vi "XYZ Stage Driver.vi"(11 "UI elements cluster":T1) -> (0 "error out (no error)":errorcluster)   [LabVIEW 2013]
uses:
  Typedefs/XYZ stage states.ctl
  Typedefs/UI ctrl refs cluster.ctl
  Typedefs/Laser control knob.ctl
  Typedefs/Frame Size.ctl
  Typedefs/Plane Mode.ctl
  Typedefs/PMT control knob.ctl
  Typedefs/HW config states enum.ctl
  Globals/gl_XYZStage globals.vi
  Global Variables/General Globals.vi
  Global Variables/gl_UI Ctrl Refs.vi
panel:
  out "Command":T2
  out "Coordinates":cluster{"X":sgl, "Y":sgl, "Z":sgl}
  out "internal error cluster":errorcluster
  # "XYZ STAGE DRIVER"
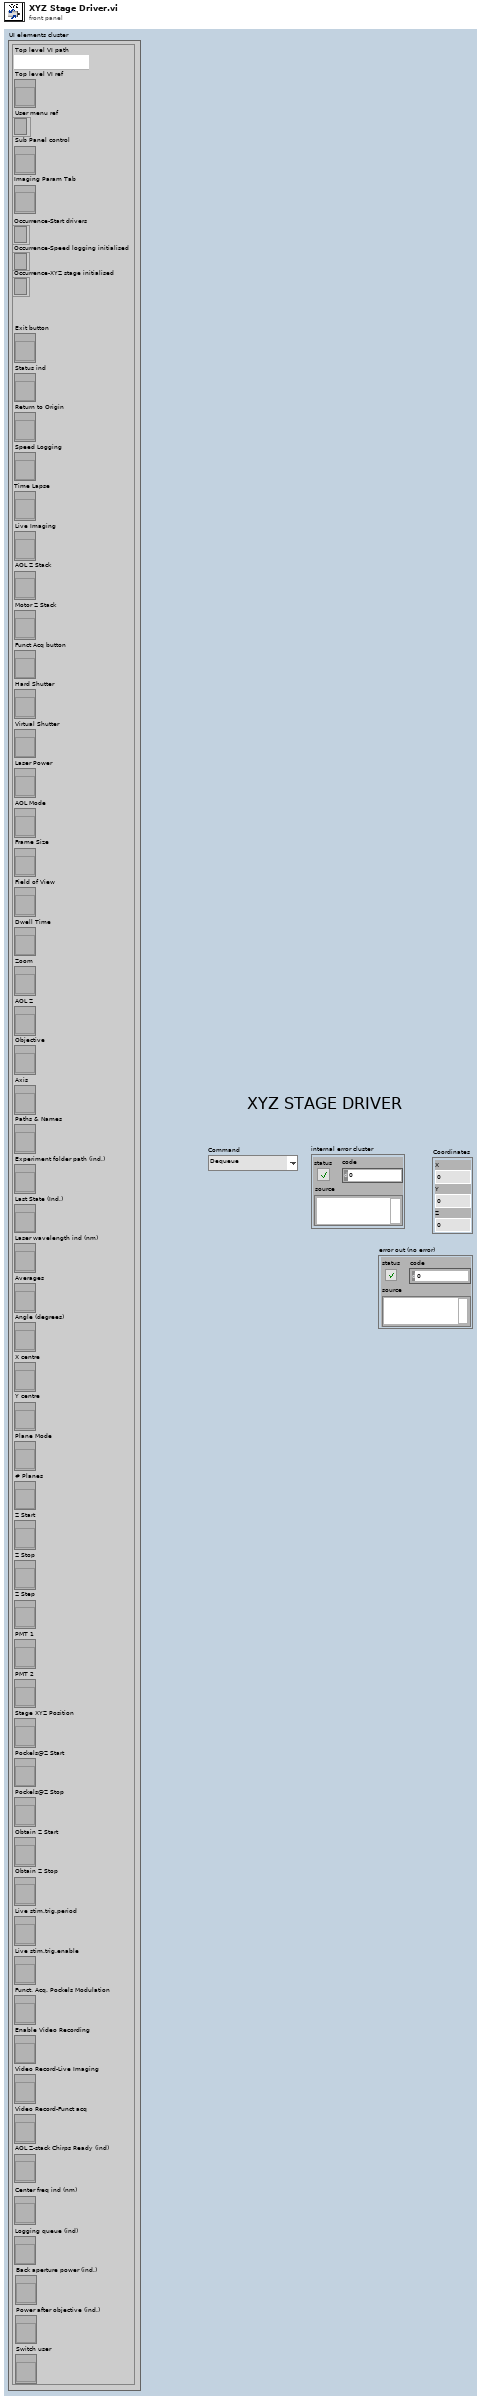
[diagram p1: front panel]
types:
  T1 = typedef "UI ctrl refs cluster.ctl" = cluster{"Top level VI path":path, "Top level VI ref":refnum<vi>, "User menu ref":refnum<k9>, "Sub Panel control":refnum<vi>, "Imaging Param Tab":refnum<vi>, "Occurrence-Start drivers":refnum<k4>, "Occurrence-Speed logging initialised":refnum<k4>, "Occurrence-XYZ stage initialised":refnum<k4>, "Exit button":refnum<vi>, "Status ind":refnum<vi>, "Return to Origin":refnum<vi>, "Speed Logging":refnum<vi>, "Time Lapse":refnum<vi>, "Live Imaging":refnum<vi>, "AOL Z Stack":refnum<vi>, "Motor Z Stack":refnum<vi>, "Funct Acq button":refnum<vi>, "Hard Shutter":refnum<vi>, "Virtual Shutter":refnum<vi>, "Laser Power":refnum<vi>, "AOL Mode":refnum<vi>, "Frame Size":refnum<vi>, "Field of View":refnum<vi>, "Dwell Time":refnum<vi>, "Zoom":refnum<vi>, "AOL Z":refnum<vi>, "Objective":refnum<vi>, "Axis":refnum<vi>, "Paths & Names":refnum<vi>, "Experiment folder path (ind.)":refnum<vi>, "Last State (Ind.)":refnum<vi>, "Laser wavelength ind (nm)":refnum<vi>, "Averages":refnum<vi>, "Angle (degrees)":refnum<vi>, "X centre":refnum<vi>, "Y centre":refnum<vi>, "Plane Mode":refnum<vi>, "# Planes":refnum<vi>, "Z Start":refnum<vi>, "Z Stop":refnum<vi>, "Z Step":refnum<vi>, "PMT 1":refnum<vi>, "PMT 2":refnum<vi>, "Stage XYZ Position":refnum<vi>, "Pockels@Z Start":refnum<vi>, "Pockels@Z Stop":refnum<vi>, "Obtain Z Start":refnum<vi>, "Obtain Z Stop":refnum<vi>, "Live stim.trig.period":refnum<vi>, "Live stim.trig.enable":refnum<vi>, "Funct. Acq. Pockels Modulation":refnum<vi>, "Enable Video Recording":refnum<vi>, "Video Record-Live Imaging":refnum<vi>, "Video Record-Funct acq":refnum<vi>, "AOL Z-stack Chirps Ready (ind)":refnum<vi>, "Center freq ind (nm)":refnum<vi>, "Logging queue (ind)":refnum<vi>, "Back aperture power (ind.)":refnum<vi>, "Power after objective (ind.)":refnum<vi>, "Switch user":refnum<vi>}
  T2 = typedef "XYZ stage states.ctl" = enum16{"Dequeue", "Initialize", "Read Position", "Read Speed Setting", "Move", "Set Max Speed", "Reset Axis", "Stop all movement"}
  T3 = typedef "HW config states enum.ctl" = enum16{"Load from file", "Save to file", "Write all", "Read all", "Write XY stage settings", "Write DAQ FPGA settings", "Write Control FPGA settings", "Write Phys Channels", "Clear", "Compare from file"}
  T4 = typedef "Sys Configuration.ctl" = cluster{"XY Stage":T5, "DAQ FPGA":T6, "Control system":T10, "Encoder":T11, "DAQmx Chan":T12, "Computer MAC address":string, "Cam VidRec":T13, "Externalise Triggers":bool, "Laser wavelength (nm)":dbl}
  T5 = typedef "XY Stage config cluster.ctl" = cluster{"COM port":refnum<visa-resource-name>, "XY stage available":bool}
  T6 = typedef "DAQ FPGA config cluster.ctl" = cluster{"Ref":T7, "Target":T8, "Clock Freq (MHz) ":dbl, "input card type":T9, "Samples Wait after Trigger":u16, "AOD fill":u16, "StartupDelay":i32, "Slip Cycle (clock cycles)":u32, "Add Cycle":bool}
  T7 = typedef "FPGA Ref.ctl" = refnum<k20>
  T8 = typedef "nirio_resource_hc.ctl" = tag
  T9 = typedef "FPGA input type AC-DC.ctl" = enum16{"AC Card", "DC Card"}
  T10 = typedef "CTRL system config cluster.ctl" = cluster{"Ethernet opened":bool, "Ethernet Port":u32, "Ctrl FPGA available":bool, "Ctrl FPGA Clock (MHz)":dbl, "Ctrl system MAC address":string, "Control system.Network adapter name":string, "AOD 1 Amplitude":i16, "AOD 2 Amplitude":i16, "AOD 3 Amplitude":i16, "AOD 4 Amplitude":i16, "Data Time Interval (ns)":dbl, "T0 (ns)":dbl, "Ta (ns)":dbl}
  T11 = typedef "Encoder config cluster.ctl" = cluster{"IP address":string, "Port":u16, "Encoder available":bool, "Wheel radius (cm)":dbl}
  T12 = typedef "DAQmx physical channels cluster.ctl" = cluster{"Pockels AO":tag, "Hard shutter AO":tag, "PMT AOs":tag, "Power meter AI":tag}
  T13 = typedef "Cam VidRec HW config setup cluster.ctl" = cluster{"DO flag-Video record":tag, "DO flag-Trial start":tag, "VidRec available":bool}
  T14 = typedef "XYZ stage data.ctl" = cluster{"Command":T2, "Channel":T15, "X":sgl, "Y":sgl, "Z":sgl, "Speed":i32, "Zero":bool, "Use acknowledgement?":bool}
  T15 = typedef "XYZ channel ring.ctl" = string
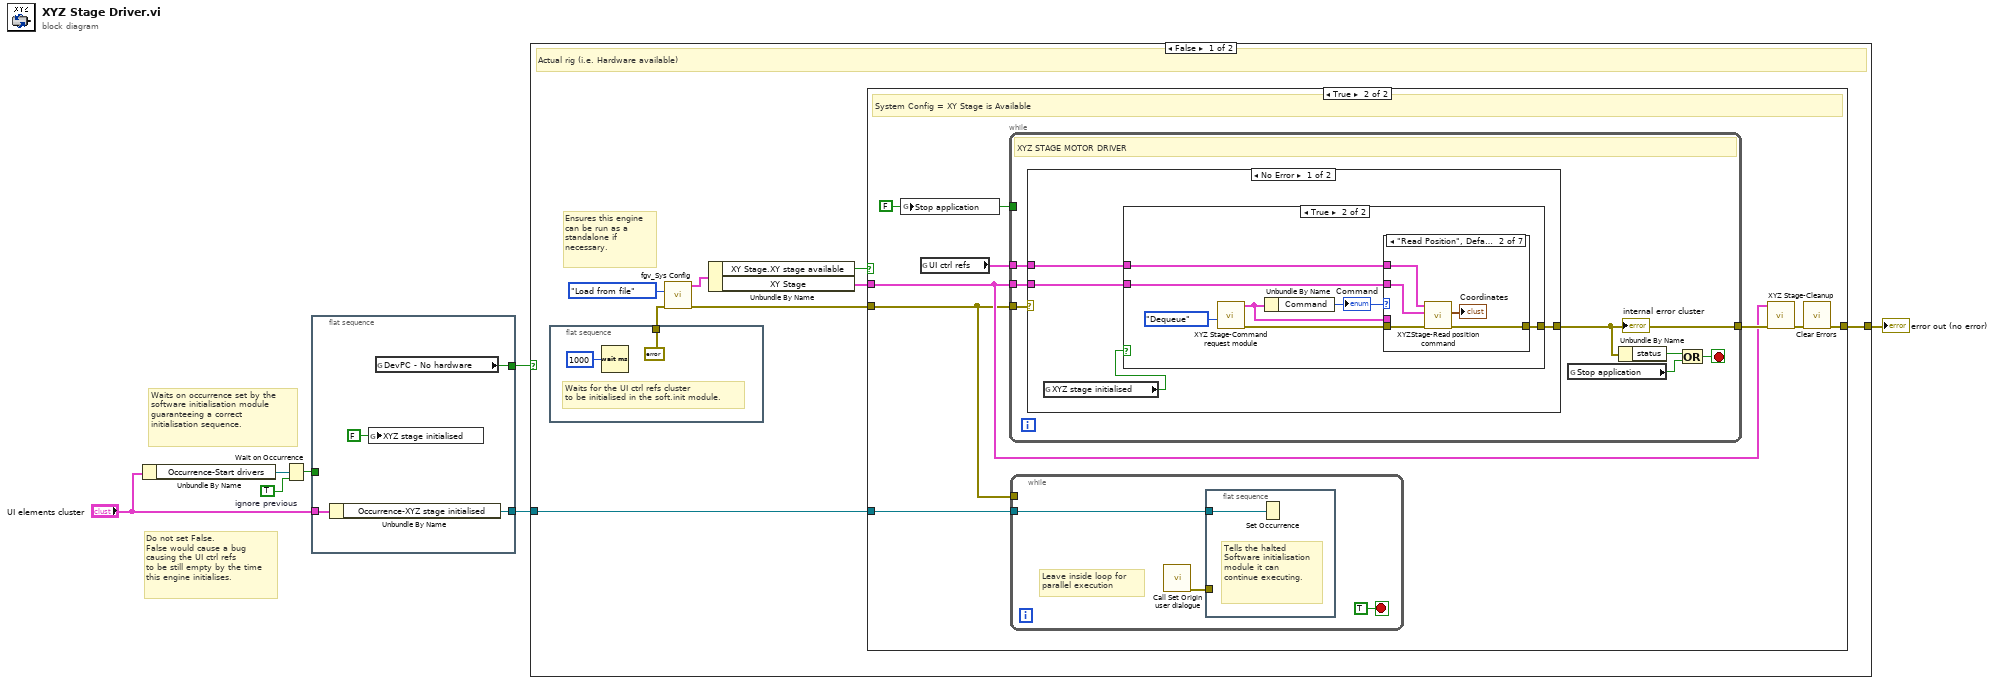
[diagram p0: block diagram]
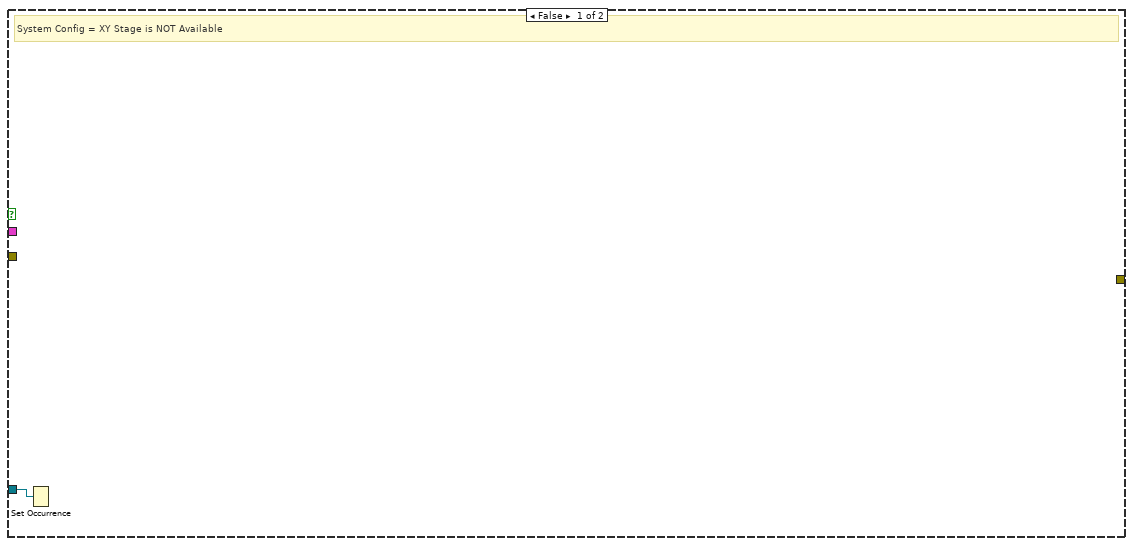
[diagram p2: hidden frame]
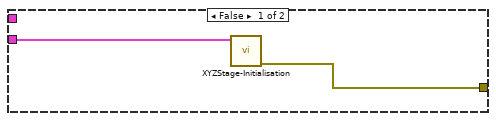
[diagram p3: hidden frame]
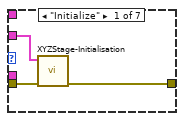
[diagram p4: hidden frame]
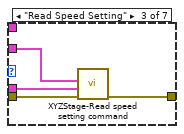
[diagram p5: hidden frame]
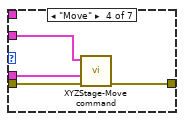
[diagram p6: hidden frame]
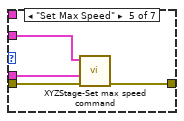
[diagram p7: hidden frame]
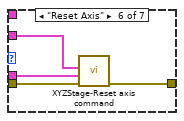
[diagram p8: hidden frame]
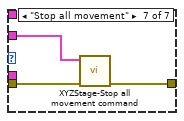
[diagram p9: hidden frame]
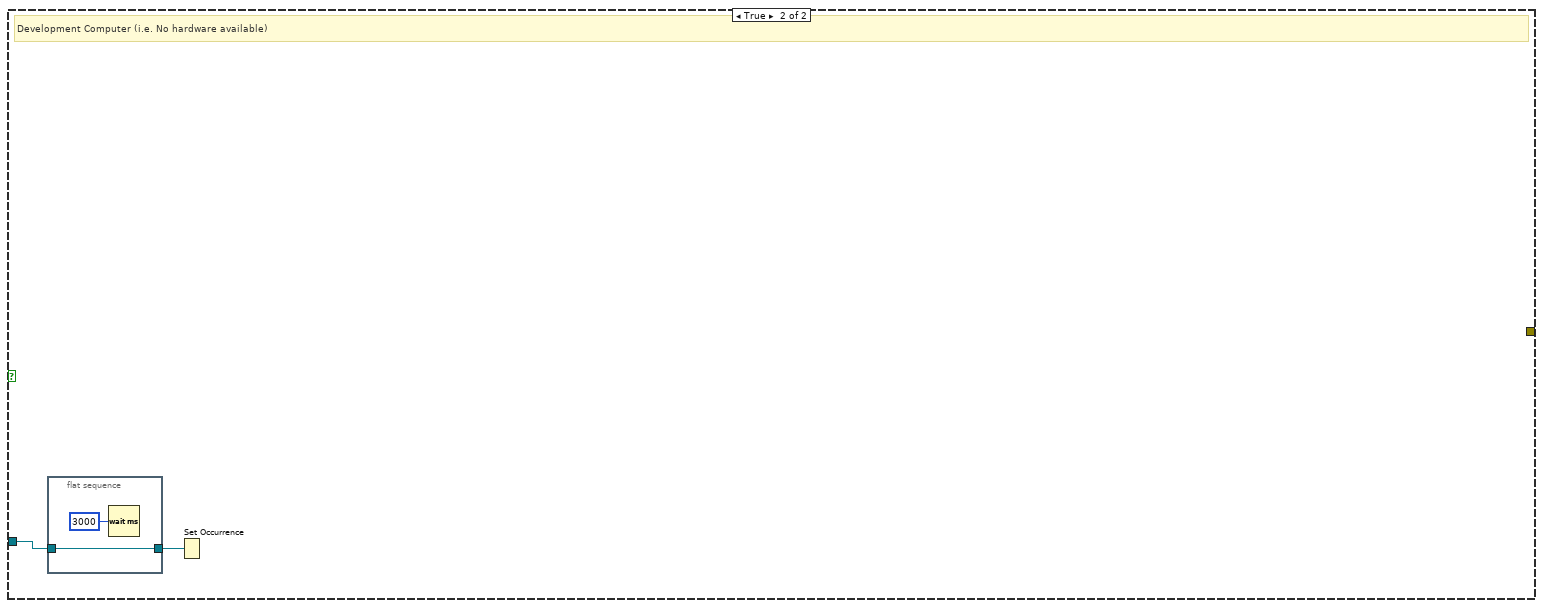
[diagram p11: hidden frame]
diagram:
  w3 = TRUE  # ignore previous
  # "Do not set False.\nFalse would cause a bug\ncausing the UI ctrl refs\nto be still empty by the time\nthis engine initialises."
  # "Waits on occurrence set by the software initialisation module guaranteeing a correct initialisation sequence."
  n1 = Unbundle By Name("UI elements cluster") -> ("Occurrence-Start drivers"=w2:refnum<k4>)
  n2 = Wait on Occurrence(1:w3, 2:w2) -> (0:w1:bool)  [unwired: 1 in]
  n3 = flat-sequence {
    tunnel: [w11] -> w6
    tunnel: "UI elements cluster" -> [w10]
    tunnel: [w9] -> w5
    tunnel: w1 -> [_]
    frame #0 {
      n4 = Unbundle By Name(w10) -> ("Occurrence-XYZ stage initialised"=w9:refnum<k4>)
      n5 = global write "gl_XYZStage globals.vi" "XYZ stage initialised"(FALSE ("XYZ stage initialised")) -> ()
      n6 = global read "General Globals.vi" "DevPC - No hardware"() -> (w11:bool)
    }
  }
  n7 = case shown="False" w6 {
    tunnel: [w15 _] -> w7
    tunnel: w5 -> [w12 w84]
    frame False {
      # "Ensures this engine can be run as a standalone if necessary."
      # "Actual rig (i.e. Hardware available)"
      n8 = flat-sequence {
        tunnel: [errorcluster {"status"=FALSE, "code"=0, "source"=""} ("error in (no error)")] -> w13
        frame #0 {
          # "Waits for the UI ctrl refs cluster\nto be initialised in the soft.init module."
          n9 = Wait (ms)(milliseconds to wait=u32 1000) -> ()  [unwired: 1 out]
        }
      }
      n10 = call "fgv_Sys Config.vi"("error in (no error)"=w13, "Function"=HW_config_states_enum."Load from file") -> ("error out"=w16:errorcluster, "System Config out"=w17:T4)  [unwired: 8 in]
      n11 = Unbundle By Name(w17) -> ("XY Stage.XY stage available"=w14:bool, "XY Stage"=w19:T5)
      n12 = case shown="True" w14 {
        tunnel: w19 -> [_ w29]
        tunnel: w12 -> [w22 w28]
        tunnel: w16 -> [_ w26]
        tunnel: [_ w24] -> w15
        frame False {
          # "System Config = XY Stage is NOT Available"
          n13 = Set Occurrence(w22) -> ()
        }
        frame True {
          w27 = FALSE ("Stop application")
          # "System Config = XY Stage is Available"
          n14 = global write "General Globals.vi" "Stop application"(w27) -> ()
          n15 = global read "gl_UI Ctrl Refs.vi" "UI ctrl refs"() -> (w23:T1)
          n16 = while {
            tunnel: w26 -> [w38]
            tunnel: [w36] -> w30
            tunnel: w29 -> [w39]
            tunnel: w27 -> [_]
            tunnel: w23 -> [w35]
            stop <- w41 stop-if-true
            # "XYZ STAGE MOTOR DRIVER"
            n17 = case shown="No Error" w38 {
              selector: w38 -> [_ w82]
              tunnel: [w44 w82] -> w36
              tunnel: w39 -> [w45 _]
              tunnel: w35 -> [w42 _]
              frame No Error {
                n18 = global read "gl_XYZStage globals.vi" "XYZ stage initialised"() -> (w43:bool)
                n19 = case shown="True" w43 {
                  tunnel: w45 -> [w47 w54]
                  tunnel: [w46 w53] -> w44
                  tunnel: w42 -> [_ w48]
                  frame False {
                    n20 = call "XYZStage-Initialisation.vi"("XY Stage"=w47) -> ("Error Out"=w46:errorcluster)  [unwired: 9 in, 1 out]
                  }
                  frame True {
                    n21 = call "XYZ Stage-Command request module.vi"("Command"=XYZ_stage_states."Dequeue") -> ("error out"=w51:errorcluster, "XYZ Stage dequeued data"=w50:T14)  [unwired: 6 in, 3 out]
                    n22 = Unbundle By Name(w50) -> ("Command"=w52:T2)
                    "Command" <- w52
                    n23 = case shown="\"Read Position\", Default" w52 {
                      tunnel: w54 -> [w56 w61 w66 w68 w72 w78 w79]
                      tunnel: w50 -> [_ _ w63 w67 w71 w75 _]
                      tunnel: w51 -> [w57 w62 w65 w70 w74 w76 w80]
                      tunnel: [w55 w60 w64 w69 w73 w77 w81] -> w53
                      tunnel: w48 -> [_ w58 _ _ _ _ _]
                      frame "Initialize" {
                        n24 = call "XYZStage-Initialisation.vi"("Error In"=w57, "XY Stage"=w56) -> ("Error Out"=w55:errorcluster)  [unwired: 8 in, 1 out]
                      }
                      frame "Read Position", Default {
                        n25 = call "XYZStage-Read position command.vi"("error in (no error)"=w62, "XY Stage config cluster"=w61, "UI ctrl refs"=w58) -> ("error out"=w60:errorcluster, "Coordinates"=→"Coordinates":cluster{"X":sgl, "Y":sgl, "Z":sgl})  [unwired: 7 in]
                      }
                      frame "Read Speed Setting" {
                        n26 = call "XYZStage-Read speed setting command.vi"("error in (no error)"=w65, "XYZ Stage data to queue"=w63, "XY Stage config cluster"=w66) -> ("error out"=w64:errorcluster)  [unwired: 8 in]
                      }
                      frame "Move" {
                        n27 = call "XYZStage-Move command.vi"("Error In"=w70, "XYZ Stage data"=w67, "XYZ Stage config"=w68) -> ("Error Out"=w69:errorcluster)  [unwired: 7 in, 1 out]
                      }
                      frame "Set Max Speed" {
                        n28 = call "XYZStage-Set max speed command.vi"("Error In"=w74, "XYZ Stage data"=w71, "XYZ Stage config"=w72) -> ("Error Out"=w73:errorcluster)  [unwired: 8 in]
                      }
                      frame "Reset Axis" {
                        n29 = call "XYZStage-Reset axis command.vi"("error in (no error)"=w76, "XYZ Stage dequeued data"=w75, "XY Stage"=w78) -> ("error out"=w77:errorcluster)  [unwired: 8 in]
                      }
                      frame "Stop all movement" {
                        n30 = call "XYZStage-Stop all movement command.vi"("Error In"=w80, "XYZ Stage config"=w79) -> ("Error Out"=w81:errorcluster)  [unwired: 8 in, 1 out]
                      }
                    }
                  }
                }
              }
              frame Error {
              }
            }
            "internal error cluster" <- w36
            n31 = global read "General Globals.vi" "Stop application"() -> (w37:bool)
            n32 = Unbundle By Name(w36) -> ("status"=w40:bool)
            n33 = Compound Arithmetic op=OR(w40, w37) -> (w41:bool)
          }
          n34 = while {
            tunnel: w26 -> [_]
            tunnel: w28 -> [w31]
            stop <- TRUE stop-if-true
            # "Leave inside loop for parallel execution"
            n35 = call "Call Set Origin user dialogue.vi"() -> ("error out"=w32:errorcluster)  [unwired: 11 in]
            n36 = flat-sequence {
              tunnel: w32 -> [_]
              tunnel: w31 -> [w34]
              frame #0 {
                # "Tells the halted Software initialisation\nmodule it can continue executing."
                n37 = Set Occurrence(w34) -> ()
              }
            }
          }
          n38 = call "XYZ Stage-Cleanup.vi"("error in (no error)"=w30, "XY Stage config cluster"=w29) -> ("error out"=w25:errorcluster)  [unwired: 9 in]
          n39 = call <vilib>:"Clear Errors.vi"("error in (no error)"=w25) -> ("error out"=w24:errorcluster)  [unwired: 6 in]
        }
      }
    }
    frame True {
      # "Development Computer (i.e. No hardware available)"
      n40 = flat-sequence {
        tunnel: w84 -> [w86]
        tunnel: [w86] -> w83
        frame #0 {
          n41 = Wait (ms)(milliseconds to wait=u32 3000) -> ()  [unwired: 1 out]
        }
      }
      n42 = Set Occurrence(w83) -> ()
    }
  }
  "error out (no error)" <- w7
